vi "Set Multipliers (no wait).vi"(7 "new mult":dbl, 11 "error in (no error)":errorcluster) -> (15 "error out":errorcluster={"status"=FALSE, "code"=0, "source"="."})   [LabVIEW 2015]
uses:
  PXI Globals.vi
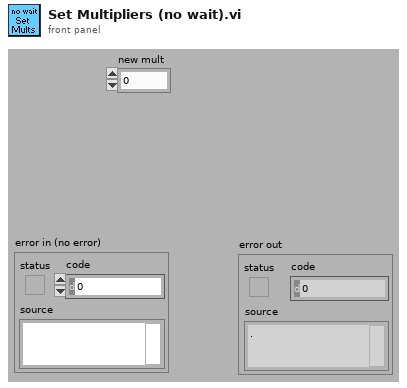
[diagram p1: front panel]
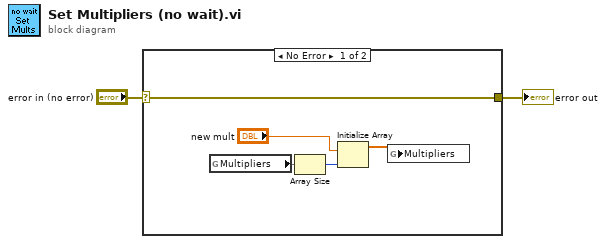
[diagram p0: block diagram]
diagram:
  n1 = case shown="No Error" "error in (no error)" {
    selector: "error in (no error)" -> [w3 w8]
    tunnel: [w3 w8] -> w1
    frame No Error {
      n2 = global read "PXI Globals.vi" "Multipliers"() -> (w7)
      n3 = Array Size(array=w7) -> (size(s)=w6:i32)
      n4 = Initialize Array("new mult", w6) -> (w5:dbl[])
      n5 = global write "PXI Globals.vi" "Multipliers"(w5) -> ()
    }
    frame Error {
    }
  }
  "error out" <- w1
